vi "FM_Receiver.vi"() -> ()   [LabVIEW 2020]
uses:
  <vilib>/sound2/lvsound2.llb/Sampling Mode.ctl
  <vilib>/sound2/lvsound2.llb/Sound Data Format.ctl
  <vilib>/Analysis/2dsp.llb/Complex FFT.vi
  HackRF_Lib/HackRF_Read_Complex.vi
  <vilib>/measure/maresamp.llb/Resample Waveform (single shot).vi
  <vilib>/sound2/lvsound2.llb/Sound Output Write (DBL Single).vi
  <vilib>/sound2/lvsound2.llb/Sound Output Set Volume (Single).vi
  <vilib>/measure/NI_MAPro.lvlib
  <vilib>/Analysis/NI_AALPro.lvlib
panel:
  out "FFT":cluster{"f0":dbl, "df":dbl, "magnitude":dbl[]}[](graph)=[{"f0"=99796744.57429048, "df"=20.0, "magnitude"=array[225000 elements]}, {"f0"=100103505.84307179, "df"=1.0, "magnitude"=[0.0, 10000000.0]}, {"f0"=101505843.07178631, "df"=1.0, "magnitude"=[0.0, 10000000.0]}, {"f0"=102106844.74123539, "df"=1.0, "magnitude"=[0.0, 10000000.0]}, {"f0"=102707846.41068447, "df"=1.0, "magnitude"=[0.0, 10000000.0]}, {"f0"=102988313.85642737, "df"=1.0, "magnitude"=[0.0, 10000000.0]}, {"f0"=104110183.63939899, "df"=1.0, "magnitude"=[0.0, 10000000.0]}]
  in  "Tuner":dbl(slide)=102046744.57429048 scale=86000000.0..110000000.0 scale format="%#_6p"
  in  "Stations":cluster{"Station":dbl, "Volume":dbl}[](array[cluster])=[{"Station"=100103505.84307179, "Volume"=0.0}, {"Station"=101505843.07178631, "Volume"=0.0}, {"Station"=102106844.74123539, "Volume"=0.4444444444444445}, {"Station"=102707846.41068447, "Volume"=0.0}, {"Station"=102988313.85642737, "Volume"=0.0}, {"Station"=104110183.63939899, "Volume"=0.0}] {"Volume" scale=0.0..1.0; "Station" scale=86000000.0..110000000.0 scale format="%#_6p"}
  out "Audio":waveform(dbl)(graph)={"t0"=timestamp(0 s since 1904-01-01), "dt"=2.2675736961451248e-05, "Y"=array[2205 elements]}
  in  "FilterFreq":dbl=3000000.0 format="%#_6p"
  in  "SampleFreq":dbl=4500000.0 format="%#_6p"
  in  "VGAGainDb":dbl=40.0 min=0.0 max=62.0 step=2.0
  in  "LNAGainDb":dbl=24.0 min=0.0 max=40.0 step=8.0
  in  "AMPEnable":bool=TRUE
  in  "Amplifier":dbl(knob)=1.2380352176045968 scale=0.01..100.0
  in  "Volume":dbl(slide)=80.61224489795919 scale=0.0..100.0
  in  "stop":bool
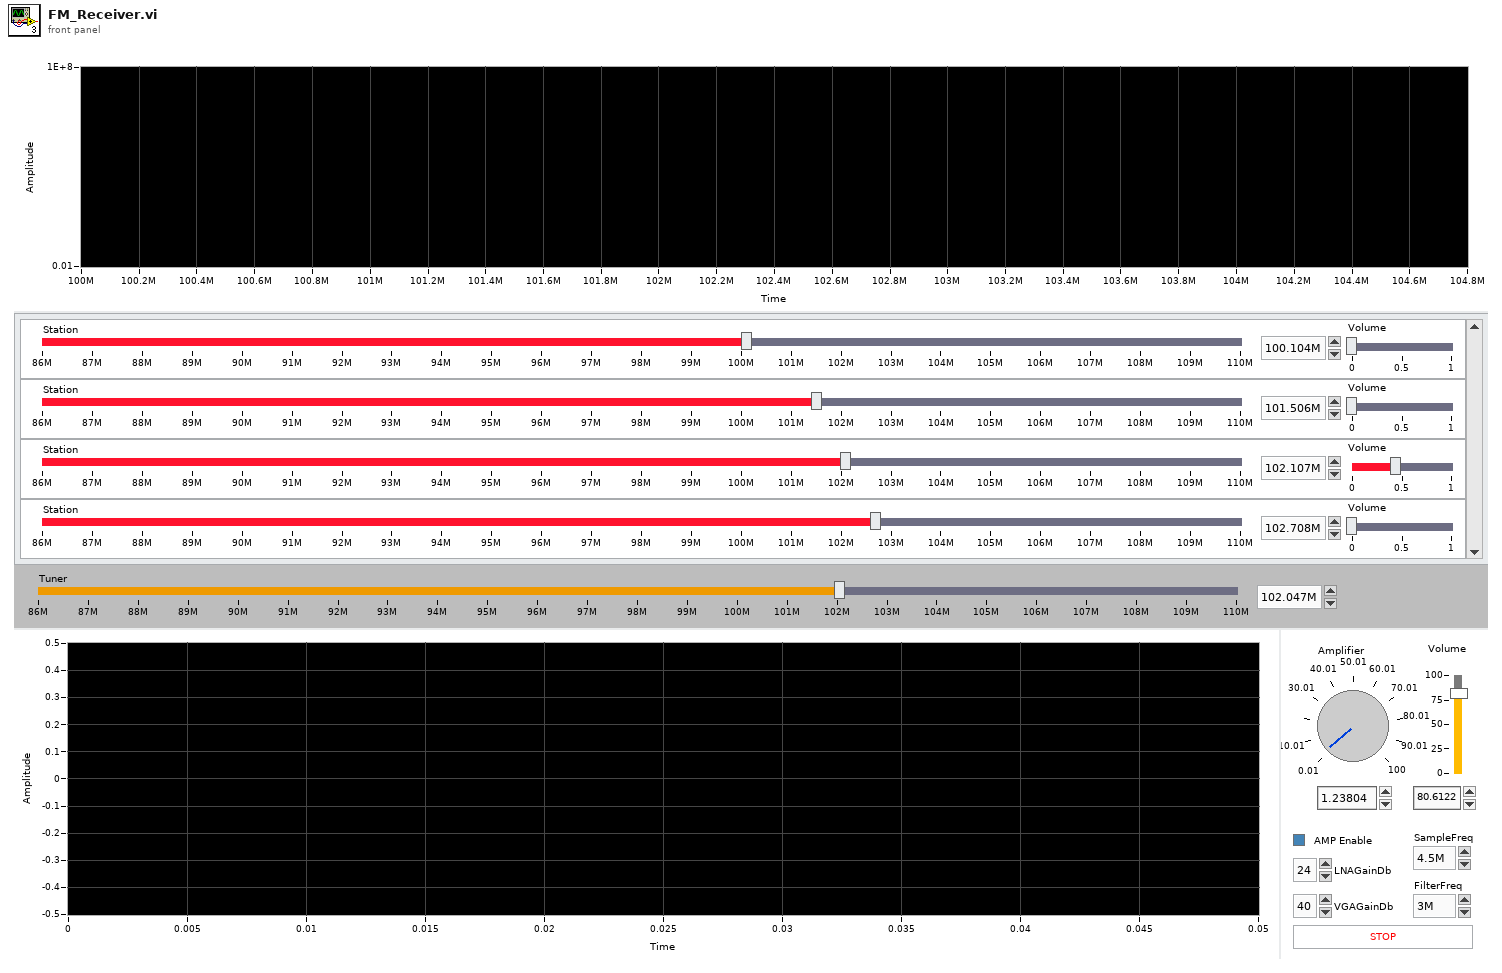
[diagram p1: front panel]
types:
  T1 = typedef "Sound Data Format.ctl" = cluster{"sample rate (S/s)":dbl, "number of channels":i32, "bits per sample":i32}
  T2 = typedef "Sampling Mode.ctl" = i32
  T3 = typedef "Sound Output Task ID.ctl" = u32
  T4 = typedef "HackRF_Ref.ctl" = cluster{".net":refnum<k24>, "HackrfDeviceList":refnum<k24>[], "OpenDevice":refnum<k24>, "StartRX":refnum<k24>, "CarrierFreqHz":dbl, "SampleFreqHz":dbl, "FilterBandwidthHz":dbl, "AMPEnable":bool, "LNAGainDb":dbl, "VGAGainDb":dbl, "StartTx":refnum<k24>}
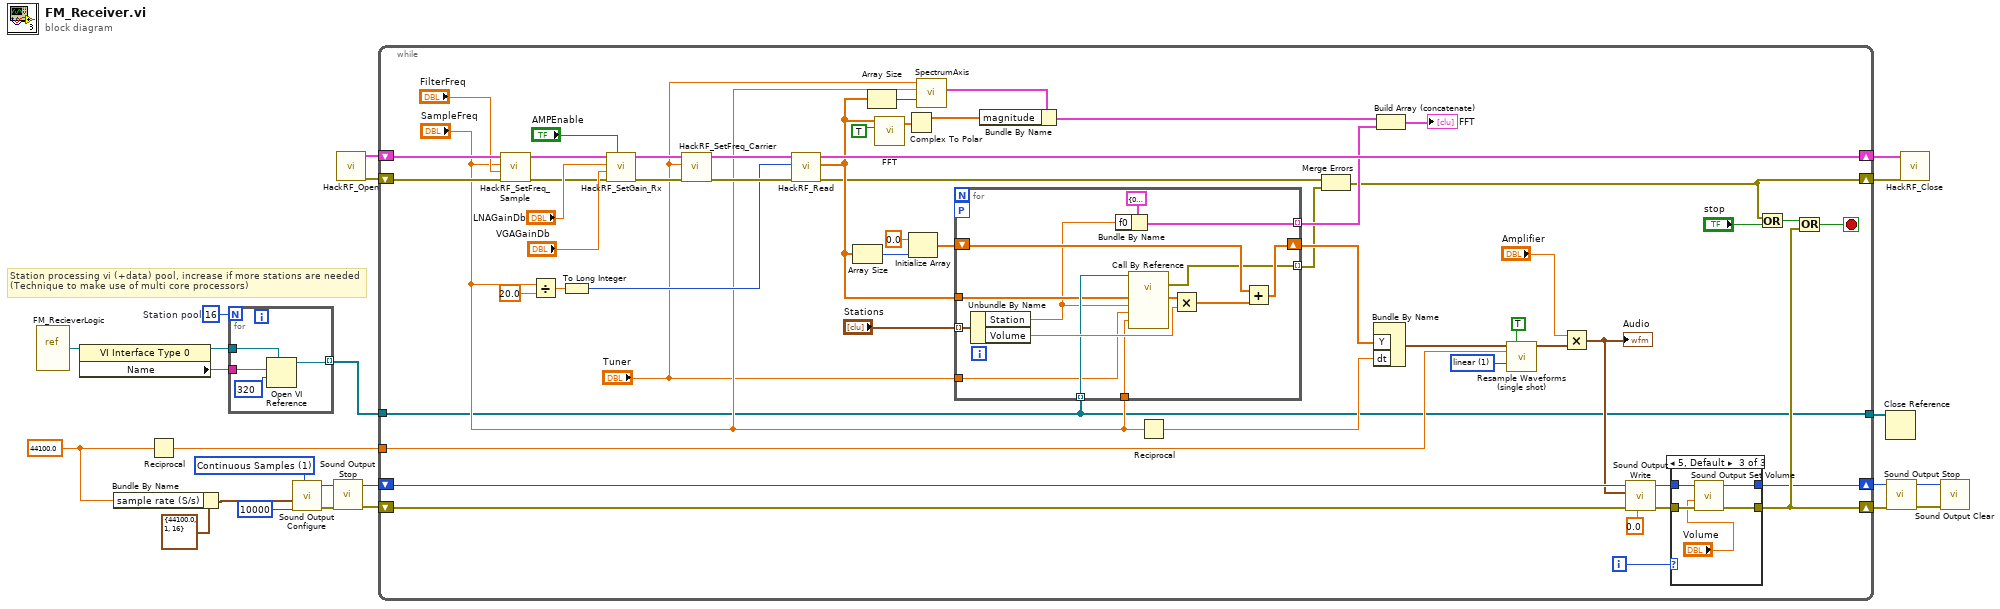
[diagram p0: block diagram]
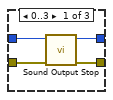
[diagram p2: hidden frame]
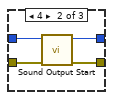
[diagram p3: hidden frame]
diagram:
  w3 = 16  # Station pool
  w17 = 44100.0 ("dt")
  w22 = T2 1 items=["Finite Samples", "Continuous Samples"] ("sample mode")
  # "Station processing vi (+data) pool, increase if more stations are needed\n(Technique to make use of multi core processors)"
  n1 = vi-ref "FM_RecieverLogic.vi"() -> (w6:refnum<vi>)
  n2 = property class="VI Interface Type 0"(reference=w6) -> (reference out=w4:refnum<vi>, "Name"=w5:string)  [unwired: 1 in, 1 out]
  n3 = Bundle By Name(cluster=T1 {"sample rate (S/s)"=44100.0, "number of channels"=1, "bits per sample"=16} ("sound format"), "sample rate (S/s)"=w17) -> (w16:T1)
  n4 = Reciprocal(x=w17) -> (1/x=w21:dbl)
  n5 = for {
    N: w3 -> [_]
    tunnel: w5 -> [w28]
    tunnel: w4 -> [w27]
    tunnel: [w25] -> w2 mode=indexing
    n6 = Open VI Reference(type specifier VI Refnum (for type only)=w27, vi path=w28, options=320) -> (vi reference=w25:refnum<vi>)  [unwired: 3 in, 1 out]
  }
  n7 = call <vilib>:"Sound Output Configure.vi"("number of samples/ch"=10000, "sample mode"=w22, "sound format"=w16) -> ("error out"=w13:errorcluster, "task ID"=w12:T3)  [unwired: 7 in]
  n8 = call <vilib>:"Sound Output Stop.vi"("error in (no error)"=w13, "task ID"=w12) -> ("error out"=w15:errorcluster, "task ID out"=w14:T3)  [unwired: 8 in]
  n9 = call "HackRF_Open.vi"() -> ("error out"=w8:errorcluster, "Cluster"=w7:T4)  [unwired: 10 in]
  n10 = while {
    shift-right: [w30] -> w24
    shift-left: w8 -> [w50]
    shift-right: [w83] -> w23
    shift-left: w7 -> [w47]
    shift-right: [w77] -> w11
    shift-left: w15 -> [w75]
    shift-right: [w76] -> w10
    shift-left: w14 -> [w74]
    tunnel: w21 -> [w56]
    tunnel: w2 -> [w29]
    tunnel: [w29] -> w1
    i -> [w73]
    stop <- w78 stop-if-true
    w58 = u16 1 items=["coerce", "linear", "spline", "FIR filter"] ("interpolation mode")
    n11 = call "HackRF_SetFreq_Sample.vi"("error in (no error)"=w50, "FilterBandwidthHz"="FilterFreq", "SampleFreqHz"="SampleFreq", "HackRF in"=w47) -> ("error out"=w49:errorcluster, "HackRF out"=w48:T4)  [unwired: 6 in]
    n12 = Divide(x="SampleFreq", y=20.0) -> (x/y=w45:dbl)
    n13 = To Long Integer(number=w45) -> (32bit integer=w43:i32)
    n14 = call "HackRF_SetGain_Rx.vi"("AMPEnable"="AMPEnable", "error in (no error)"=w49, "VGAGainDb"="VGAGainDb", "LNAGainDb"="LNAGainDb", "HackRF in"=w48) -> ("error out"=w55:errorcluster, "HackRF out"=w54:T4)  [unwired: 5 in]
    n15 = call "HackRF_SetFreq_Carrier.vi"("error in (no error)"=w55, "CarrierFreqHz"="Tuner", "HackRF_In"=w54) -> ("error out"=w80:errorcluster, "HackRF_Out"=w81:T4)  [unwired: 7 in]
    n16 = call-poly "HackRF_Read.vi"("error in (no error)"=w80, "count"=w43, "HackRF"=w81) -> ("error out"=w32:errorcluster, "Data"=w39:cdb[], "HackRF"=w83:T4)  [unwired: 6 in]
    n17 = Array Size(array=w39) -> (size(s)=w36:i32)
    n18 = Array Size(array=w39) -> (size(s)=w64:i32)
    n19 = call-poly <vilib>:"FFT.vi"("shift?"=TRUE, "X"=w39) -> ("FFT {X}"=w60:cdb[])  [unwired: 8 in, 1 out]
    n20 = Complex To Polar(r * e^(i*theta)=w60) -> (r=w62:dbl[])  [unwired: 1 out]
    n21 = Initialize Array(0.0 ("y"), w36) -> (w38:dbl[])
    n22 = call "SpectrumAxis.vi"("FFT Size"=w64, "SampleFreq"="SampleFreq", "CarrierFreqz)"="Tuner") -> ("SpectrumConstant"=w63:cluster{"f0":dbl, "df":dbl, "magnitude":dbl[]})  [unwired: 8 in]
    n23 = for {
      tunnel: w39 -> [w88]
      tunnel: "Stations" -> [w97] mode=indexing
      tunnel: "SampleFreq" -> [w85]
      tunnel: "Tuner" -> [w86]
      shift-right: [w94] -> w35
      shift-left: w38 -> [w93]
      workers-P: _ -> [_]
      tunnel: [w91] -> w34 mode=indexing
      tunnel: w29 -> [w90] mode=indexing
      tunnel: [w84] -> w31 mode=indexing
      n24 = Unbundle By Name(w97) -> ("Station"=w87:dbl, "Volume"=w96:dbl)
      n25 = Bundle By Name(cluster=cluster{"f0":dbl, "df":dbl, "magnitude":dbl[]} {"f0"=0.0, "df"=1.0, "magnitude"=[-1000.0, 10000000000.0]} ("output cluster"), "f0"=w87) -> (w91:cluster{"f0":dbl, "df":dbl, "magnitude":dbl[]})
      n26 = call-by-ref "?"(reference=w90, "SampleFrequencyHz"=w85, "Tuner in"=w86, "CarrierFrequencyHz"=w87, "Data in"=w88) -> (error out=w84:errorcluster, "Audio"=w89:dbl[])  [unwired: 7 in, 2 out]
      n27 = Multiply(x=w89, y=w96) -> (x*y=w95:dbl[])
      n28 = Add(x=w93, y=w95) -> (x+y=w94:dbl[])
    }
    n29 = Bundle By Name(cluster=w63, "magnitude"=w62) -> (w59:cluster{"f0":dbl, "df":dbl, "magnitude":dbl[]})
    n30 = Reciprocal(x="SampleFreq") -> (1/x=w42:dbl)
    n31 = Merge Errors(w32, w31) -> (w30:errorcluster)
    n32 = Bundle By Name("Y"=w35, "dt"=w42) -> (w72:waveform(dbl))  [unwired: 1 in]
    n33 = Build Array (concatenate)(w59, w34) -> (→"FFT":cluster{"f0":dbl, "df":dbl, "magnitude":dbl[]}[])
    n34 = call-poly <vilib>:"Resample Waveforms (single shot).vi"("waveform in"=w72, "open interval? (F)"=TRUE, "dt"=w56, "interpolation mode"=w58) -> ("resampled waveform out"=w68:waveform(dbl))  [unwired: 8 in, 3 out]
    n35 = Multiply(x="Amplifier", y=w68) -> (x*y=w67:waveform(dbl))
    "Audio" <- w67
    n36 = call-poly <vilib>:"Sound Output Write.vi"("timeout (sec)"=0.0, "error in (no error)"=w75, "data"=w67, "task ID"=w74) -> ("error out"=w71:errorcluster, "task ID out"=w70:T3)  [unwired: 6 in]
    n37 = case shown="5, Default" w73 {
      tunnel: w71 -> [w101 w105 w110]
      tunnel: w70 -> [w100 w104 w107]
      tunnel: [w99 w103 w109] -> w77
      tunnel: [w98 w102 w108] -> w76
      frame 0..3 {
        n38 = call <vilib>:"Sound Output Stop.vi"("error in (no error)"=w101, "task ID"=w100) -> ("error out"=w99:errorcluster, "task ID out"=w98:T3)  [unwired: 8 in]
      }
      frame 4 {
        n39 = call <vilib>:"Sound Output Start.vi"("error in (no error)"=w105, "task ID"=w104) -> ("error out"=w103:errorcluster, "task ID out"=w102:T3)  [unwired: 8 in]
      }
      frame 5, Default {
        n40 = call-poly <vilib>:"Sound Output Set Volume.vi"("error in (no error)"=w110, "volume"="Volume", "task ID"=w107) -> ("error out"=w109:errorcluster, "task ID out"=w108:T3)  [unwired: 7 in]
      }
    }
    n41 = Or(x=w30, y="stop") -> (x .or. y?=w79:bool)
    n42 = Or(x=w79, y=w77) -> (x .or. y?=w78:bool)
  }
  n43 = Close Reference(reference=w1) -> ()  [unwired: 1 in, 1 out]
  n44 = call <vilib>:"Sound Output Stop.vi"("error in (no error)"=w11, "task ID"=w10) -> ("error out"=w20:errorcluster, "task ID out"=w19:T3)  [unwired: 8 in]
  n45 = call "HackRF_Close.vi"("error in (no error)"=w24, "Cluster in"=w23) -> ()  [unwired: 8 in, 2 out]
  n46 = call <vilib>:"Sound Output Clear.vi"("error in (no error)"=w20, "task ID"=w19) -> ()  [unwired: 9 in, 1 out]
